vi "Fe Material Properties.vi"(6 "m-nm Fe":dbl, 9 "Fe Thickness":dbl, 10 "Energy (Heat; I^2R)":dbl, 11 "NS Base Area":dbl) -> (1 "Mass Fe":dbl, 2 "Delta Temp Change Fe":dbl, 3 "Fe Specfic Heat Capacity":dbl, 4 "Fe Density":dbl, 5 "Fe Thickness 2":dbl, 7 "Volume Fe":dbl)   [LabVIEW 2020]
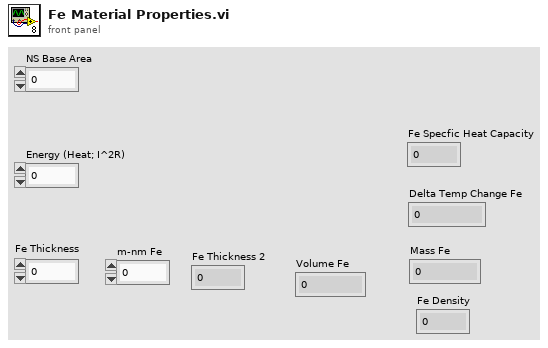
[diagram p1: front panel]
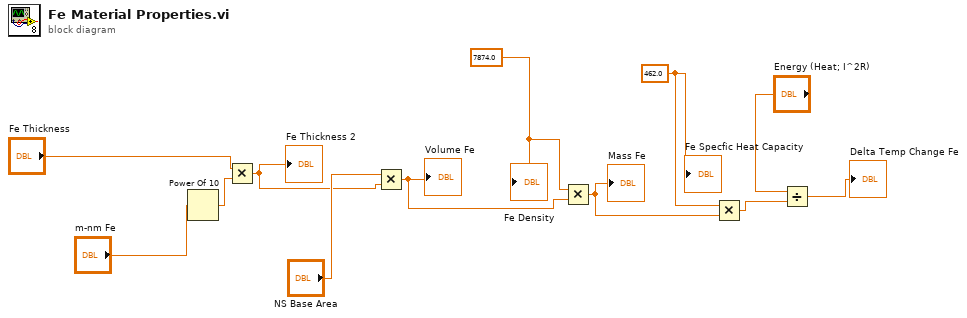
[diagram p0: block diagram]
diagram:
  w12 = 462.0 ("Silicon Specfic Heat Capacity 6")
  w5 = 7874.0 ("Silicon Density 6")
  n1 = Power Of 10(x="m-nm Fe") -> (10^x=w1:dbl)
  n2 = Multiply(x="Fe Thickness", y=w1) -> (x*y=w4:dbl)
  "Fe Thickness 2" <- w4
  n3 = Multiply(x="NS Base Area", y=w4) -> (x*y=w6:dbl)
  "Volume Fe" <- w6
  n4 = Multiply(x=w5, y=w6) -> (x*y=w11:dbl)
  "Mass Fe" <- w11
  n5 = Multiply(x=w12, y=w11) -> (x*y=w10:dbl)
  n6 = Divide(x="Energy (Heat; I^2R)", y=w10) -> (x/y=→"Delta Temp Change Fe":dbl)
  "Fe Density" <- w5
  "Fe Specfic Heat Capacity" <- w12
